vi "create TCPPacket.vi"(8 "error in (no error)":errorcluster, 9 "Encoding":T1, 10 "Content Type":T2, 11 "TCPPacket in":refnum<class "TCPPacket.lvclass">) -> (0 "error out":errorcluster, 3 "TCPPacket out":refnum<class "TCPPacket.lvclass">)   [LabVIEW 2019, in "TCPPacket.lvclass"]
uses:
  TCPPacket.lvclass
  TCPHeader ContentType STYP.ctl
  TCPHeader ContentEncoding STYP.ctl
  TCPPacket.lvclass/TCPPacket.ctl
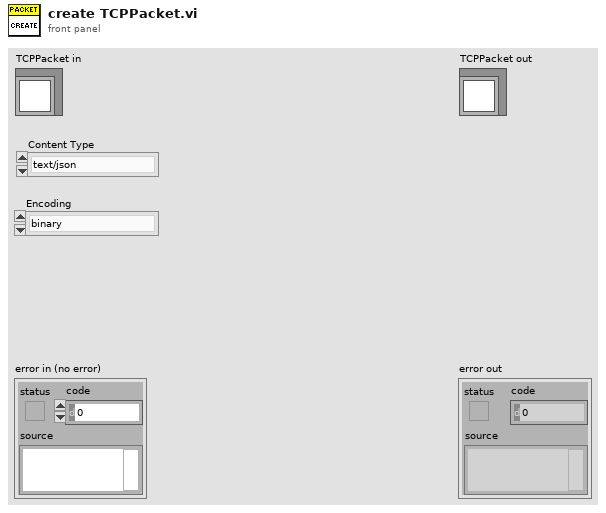
[diagram p1: front panel]
types:
  T1 = typedef "TCPPacket.lvclass/TCPHeader ContentEncoding STYP.ctl" = enum16{"binary", "utf-8", "latin-1"}
  T2 = typedef "TCPPacket.lvclass/TCPHeader ContentType STYP.ctl" = enum16{"text/json", "binary/application"}
  T3 = typedef "TCPPacket.lvclass/TCPHeader STYP.ctl" = cluster{"byteorder":string, "content-length":u32, "content-type":string, "content-encoding":string}
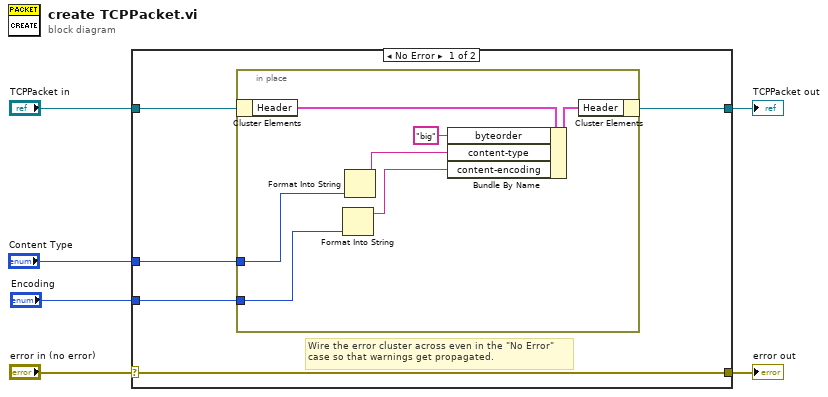
[diagram p0: block diagram]
diagram:
  n1 = case shown="No Error" "error in (no error)" {
    selector: "error in (no error)" -> [w11 w20]
    tunnel: [w11 w20] -> w5
    tunnel: [w10 w19] -> w3
    tunnel: "TCPPacket in" -> [w9 w19]
    tunnel: "Content Type" -> [w8 _]
    tunnel: "Encoding" -> [w7 _]
    frame No Error {
      # "Wire the error cluster across even in the \"No Error\"\ncase so that warnings get propagated."
      n2 = in-place {
        in-place-border: w8 -> [w16]
        in-place-border: w7 -> [w15]
        n3 = in-place-cluster #1(w9) -> ("Header"=w18:T3)
        n4 = Format Into String(w15) -> (resulting string=w13:string)  [unwired: 3 in, 1 out]
        n5 = Format Into String(w16) -> (resulting string=w14:string)  [unwired: 3 in, 1 out]
        n6 = Bundle By Name(cluster=w18, "byteorder"="big", "content-type"=w14, "content-encoding"=w13) -> (w17:T3)
        n7 = in-place-cluster #1("Header"=w17) -> (w10:refnum<class "TCPPacket.lvclass">)
      }
    }
    frame Error {
    }
  }
  "error out" <- w5
  "TCPPacket out" <- w3
